vi "Write cameras.vi"(8 "error in (no error)":errorcluster, 10 "cameras":string[](array[string]), 11 "Vision in":refnum<class "Vision.lvclass">) -> (0 "error out":errorcluster, 3 "Vision out":refnum<class "Vision.lvclass">)   [LabVIEW 2023, in "Vision.lvclass"]
uses:
  Vision.lvclass
  Vision.lvclass/Vision.ctl
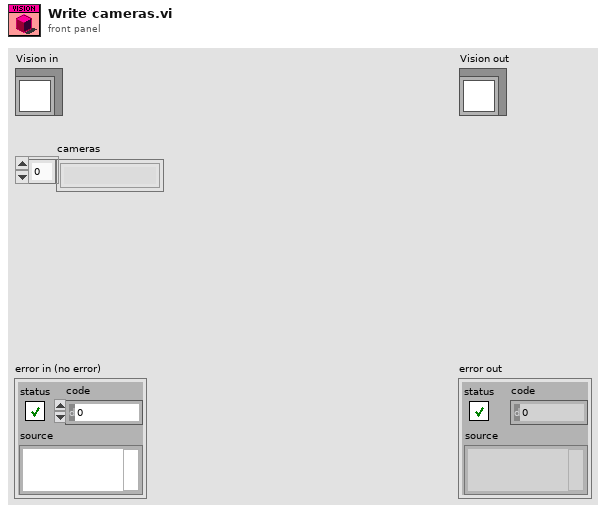
[diagram p1: front panel]
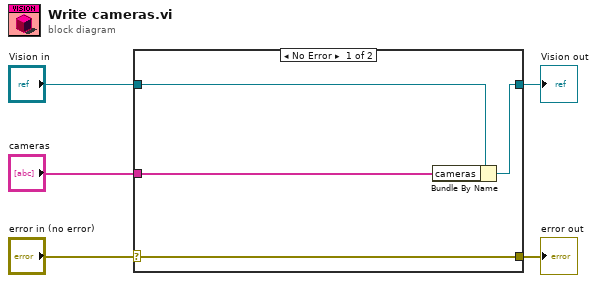
[diagram p0: block diagram]
diagram:
  n1 = case shown="No Error" "error in (no error)" {
    selector: "error in (no error)" -> [w9 w10]
    tunnel: [w9 w10] -> w4
    tunnel: [w7 w11] -> w2
    tunnel: "Vision in" -> [w8 w11]
    tunnel: "cameras" -> [w6 _]
    frame No Error {
      n2 = Bundle By Name(cluster=w8, "cameras"=w6) -> (w7:refnum<class "Vision.lvclass">)
    }
    frame Error {
    }
  }
  "error out" <- w4
  "Vision out" <- w2
